vi "Draw Body Reference Frame.vi"(2 "length":dbl=0.1, 3 "theta":dbl, 4 "Y inertial":dbl, 5 "X inertial":dbl) -> (0 "X body axis":cluster{dbl, dbl}[](array[cluster]), 1 "Y body axis":cluster{dbl, dbl}[](array[cluster]))   [LabVIEW 2011]
uses:
  <vilib>/Analysis/coordinate.llb/2D Cartesian Coordinate Rotation (Scalar).vi
  <vilib>/Analysis/NI_AALPro.lvlib
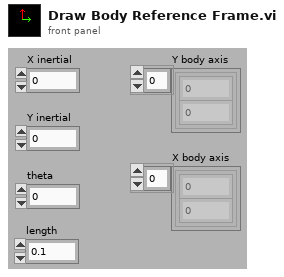
[diagram p1: front panel]
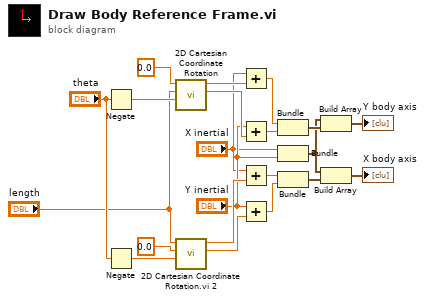
[diagram p0: block diagram]
diagram:
  n1 = Negate(x="theta") -> (-x=w7:dbl)
  n2 = Negate(x="theta") -> (-x=w19:dbl)
  n3 = call-poly <vilib>:"2D Cartesian Coordinate Rotation.vi"("theta"=w7, "y"="length", "x"=0.0) -> ("y out"=w9:dbl, "x out"=w8:dbl)  [unwired: 7 out]
  n4 = call-poly "2D Cartesian Coordinate Rotation.vi 2"("theta"=w19, "y"=0.0, "x"="length") -> ("y out"=w17:dbl, "x out"=w18:dbl)  [unwired: 7 out]
  n5 = Add(x="X inertial", y=w8) -> (x+y=w5:dbl)
  n6 = Add(x="Y inertial", y=w9) -> (x+y=w10:dbl)
  n7 = Add(x="X inertial", y=w18) -> (x+y=w16:dbl)
  n8 = Add(x="Y inertial", y=w17) -> (x+y=w15:dbl)
  n9 = Bundle(w5, w10) -> (w11:cluster{dbl, dbl})  [unwired: 1 out]
  n10 = Bundle("X inertial"="X inertial", "Y inertial"="Y inertial") -> (w2:cluster{"X inertial":dbl, "Y inertial":dbl})  [unwired: 1 out]
  n11 = Bundle(w16, w15) -> (w14:cluster{dbl, dbl})  [unwired: 1 out]
  n12 = Build Array(w2, w11) -> (→"Y body axis":cluster{"X inertial":dbl, "Y inertial":dbl}[])
  n13 = Build Array(w2, w14) -> (→"X body axis":cluster{"X inertial":dbl, "Y inertial":dbl}[])
